vi "DFD Build Filter Bank from Prototype Filter.vi"   [LabVIEW 2017, in "NI_DigFilter_FilterBank.lvlib"]
doc: "Creates a cosine-modulated filter bank from a prototype filter."
uses:
  <vilib>/addons/Digital Filter Design/NI_DigFilter_FilterBank.lvlib
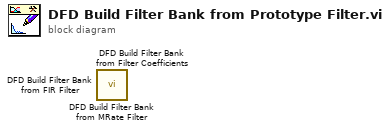
[diagram p0: block diagram]
diagram:
  n1 = call <vilib>:"DFD Build Filter Bank from MRate Filter.vi"() -> ()  [unwired: 10 in, 2 out]
  n2 = call <vilib>:"DFD Build Filter Bank from Filter Coefficients.vi"() -> ()  [unwired: 10 in, 2 out]
  n3 = call <vilib>:"DFD Build Filter Bank from FIR Filter.vi"() -> ()  [unwired: 10 in, 2 out]
